vi "Get Buffer Events.vi"(8 "error in":errorcluster, 11 "Buffer in":refnum<data-value>) -> (0 "error out":errorcluster, 2 "buffer-event":refnum<user-event>, 3 "Buffer":refnum<data-value>)   [LabVIEW 2013, in "CircularBuffer.lvlib" / "VariantBuffer.lvclass"]
doc: "This VI returns data from the ring buffer starting from the oldest data and ending with the newest.\n\nThe data is duplicated at the output so this VI allocates new place in the memory for the output."
uses:
  VariantBuffer.lvclass
  buffer-event -- enum.ctl
  VariantBuffer.lvclass/VariantBuffer.ctl
  buffer-errors -- ring.ctl
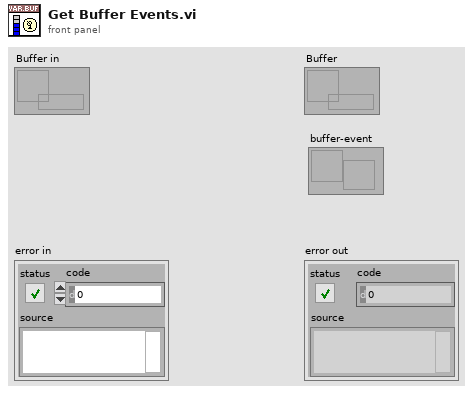
[diagram p1: front panel]
types:
  T1 = typedef "CircularBuffer.lvlib/VariantBuffer.lvclass/buffer-errors -- ring.ctl" = i32
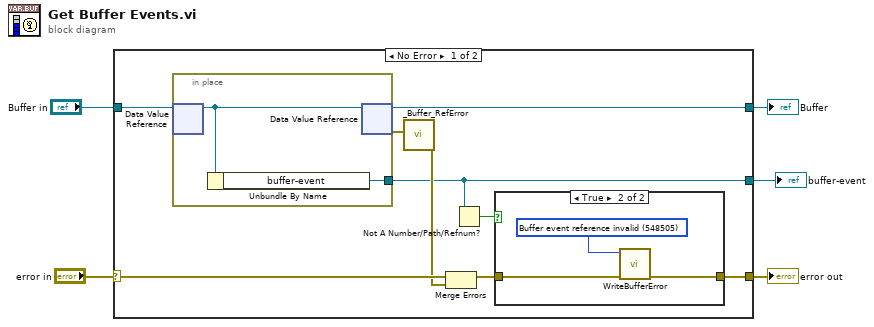
[diagram p0: block diagram]
diagram:
  n1 = case shown="No Error" "error in" {
    selector: "error in" -> [w12 w21]
    tunnel: "Buffer in" -> [w14 w22]
    tunnel: [w13 w22] -> w4
    tunnel: [w7 w21] -> w2
    tunnel: [w9 _] -> w1
    frame No Error {
      n2 = in-place {
        in-place-border: [w19] -> w9
        n3 = in-place-dvr #1(w14) -> (w20:refnum<class "VariantBuffer.lvclass">)  [unwired: 1 out]
        n4 = Unbundle By Name(w20) -> ("buffer-event"=w19:refnum<user-event>)
        n5 = in-place-dvr #1(w20) -> (w13:refnum<data-value>, w11:errorcluster)
      }
      n6 = call "_Buffer_RefError.vi"("error in (no error)"=w11) -> ("error out"=w10:errorcluster)  [unwired: 10 in]
      n7 = Merge Errors(w12, w10) -> (w6:errorcluster)
      n8 = Not A Number/Path/Refnum?(number/path/refnum=w9) -> (NaN/Path/Refnum?=w8:bool)
      n9 = case shown="True" w8 {
        tunnel: [w15 w17] -> w7
        tunnel: w6 -> [w15 w18]
        frame False {
        }
        frame True {
          w16 = T1 548505 items=["No error"=0, "Generic Buffer error"=548500, "Buffer is full"=548501, "Buffer is empty"=548502, "Buffer size cannot be 0"=548503, "Buffer reference is invalid"=548504, "Buffer event reference invalid"=548505, "Buffer Type not supported"=548506, "Not enough space in the buffer for this operation"=548507] ("buffer-errors")
          n10 = call "WriteBufferError.vi"("error in (no error)"=w18, "buffer-errors"=w16) -> ("error out"=w17:errorcluster)  [unwired: 9 in]
        }
      }
    }
    frame Error {
    }
  }
  "error out" <- w2
  "Buffer" <- w4
  "buffer-event" <- w1
